vi "mHTprofile_vector.vi"(0 "Gamma0":dbl caption="Gamma0 (0)" format="%#_13g", 1 "Delta0":dbl caption="Delta0 (0)" format="%#_13g", 2 "Gamma2":dbl caption="Gamma2 (0)" format="%#_13g", 3 "Delta2":dbl caption="Delta2 (0)" format="%#_13g", 4 "NuOptRe":dbl caption="NuOptRe (0)" format="%#_13g", 5 "NuOptIm":dbl caption="NuOptIm (0)" format="%#_13g", 6 "Xlm":dbl caption="Xlm (0)" format="%#_13g", 7 "nu0":dbl caption="nu0 (0)" format="%#_13g", 8 "Ylm":dbl caption="Ylm (0)" format="%#_13g", 9 "GammaD":dbl caption="GammaD (0)" format="%#_13g", 10 "alpha":dbl=10.0 caption="alpha (10)" format="%#_13g", 11 "nu":dbl[](array[numeric])=[0.0, 112265.43344000001, 112265.44046000001, 112265.44748000002, 112265.45450000002, 112265.46152000003, 112265.46854000003, 112265.47556000004, 112265.48258000004, 112265.48960000004, 112265.49662000005, 112265.50364000005, 112265.51066000006, 112265.51768000006, 112265.52470000007, 112265.53172000007, 112265.53874000008, 112265.54576000008, 112265.55278000009, 112265.55980000009, 112265.5668200001, 112265.5738400001, 112265.5808600001, 112265.58788000011, 112265.59490000011, 112265.60192000012, 112265.60894000012, 112265.61596000013, 112265.62298000013, 112265.63000000014, 112265.63702000014, 112265.64404000014, 112265.65106000015, 112265.65808000015, 112265.66510000016, 112265.67212000016, 112265.67914000017, 112265.68616000017, 112265.69318000018, 112265.70020000018, 112265.70722000019, 112265.71424000019, 112265.7212600002, 112265.7282800002, 112265.7353000002, 112265.74232000021, 112265.74934000021, 112265.75636000022, 112265.76338000022, 112265.77040000023, 0.0] format="%#_16g", 12 "disp":enum32{"Absorption", "Dispersion"}(ring) caption="disp (Absorption)") -> (18 "mHT":dbl[](array[numeric])=[nan, 0.10445929269462101, 0.11168038230081595, 0.11969856238844125, 0.1286377380830614, 0.13864704864655428, 0.14990727829379918, 0.16263922460671215, 0.1771147209669791, 0.19367128964614844, 0.21273180576293013, 0.23483113593592242, 0.2606525606824893, 0.29107801057316474, 0.32725789462097354, 0.3707087581774661, 0.4234503518208136, 0.4881979797546625, 0.5686309274509256, 0.6697622885290168, 0.798437386757727, 0.9639839696835227, 1.1790249509999895, 1.460444698920676, 1.8304717689294367, 2.31776489642677, 2.9580972384622766, 3.7933109622015557, 4.86494935246605, 6.194795635571412, 7.740733853926797, 9.326488123304564, 10.59710374177369, 11.127748547057859, 10.714837692264172, 9.553864870950973, 8.06020224435464, 6.58240100721215, 5.295904040882446, 4.245577585161483, 3.4134497282314253, 2.761721832470126, 2.252063531475144, 1.8520390876765764, 1.5360968914463138, 1.2847114253118193, 1.0831306600151056, 0.9202283794901738, 0.7875855185711089, 0.6787942573273069, 1.4180731455680285e-09] caption="mHT output" format="%#_16g")   [LabVIEW 2015]
panel:
  # "modified Hartman Tran profile"
  # "Subroutine to compute the complex normalized spectral-line shape using mHT model\n\nStandard Input Parameters:\n--------------------\nnu0     : Unperturbed line position in cm-1.\nGammaD  : Doppler broadening in cm-1.\nGamma0  : Speed-averaged line-width in cm-1.       \nGamma2  : Quadratic speed dependence parameter of the line-width in cm-1.\nDelta0  : Speed-averaged line-shift in cm-1.\nDelta2  : Quadratic speed dependence parameter of the line-shift in cm-1.   \nNuOptRe : Real part of the complex Dicke parameter in cm-1.\nNuOptIm : Imaginary part of the complex Dicke parameter in cm-1.    \nnu      : Current WaveNumber in cm-1.\nYlm     : Imaginary part of the 1st order (Rosenkranz) line mixing coefficients, dimensionless (default: 0.0).\nXlm     : Real part of the 1st order (Rosenkranz) line mixing coefficients, dimensionless (default: 0.0).\nalpha   : Mass ratio in the molecule for calculating beta-correction, applicable up to alpha=5, \n          dimensionless (default: 10.0).\ndisp    : Boolean trigger for including dispersion profile in the output (default: Absorption).\n\nThe function has one outputs:\n--------------------\n(1)     : Real or imaginary (depending on disp value) part of the normalized spectral shape in cm."
  # "Output Section"
  # "Input Section"
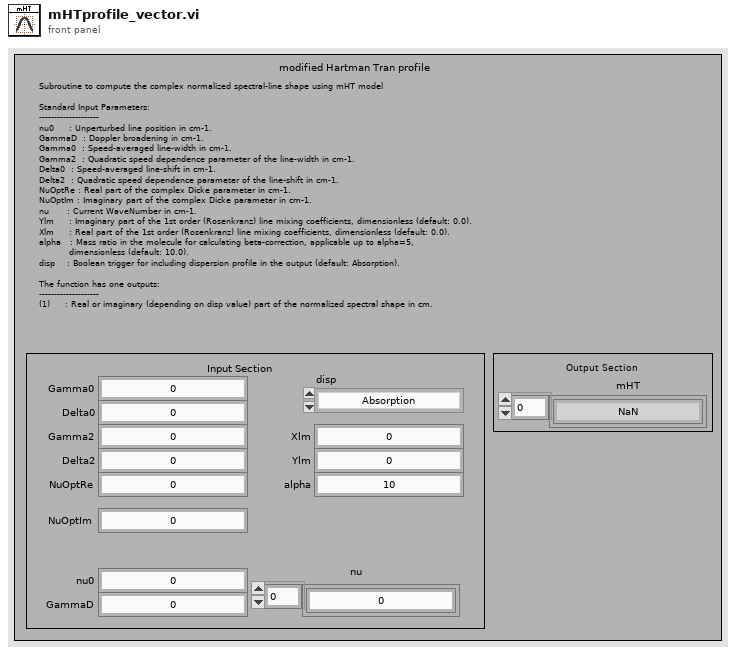
[diagram p1: front panel]
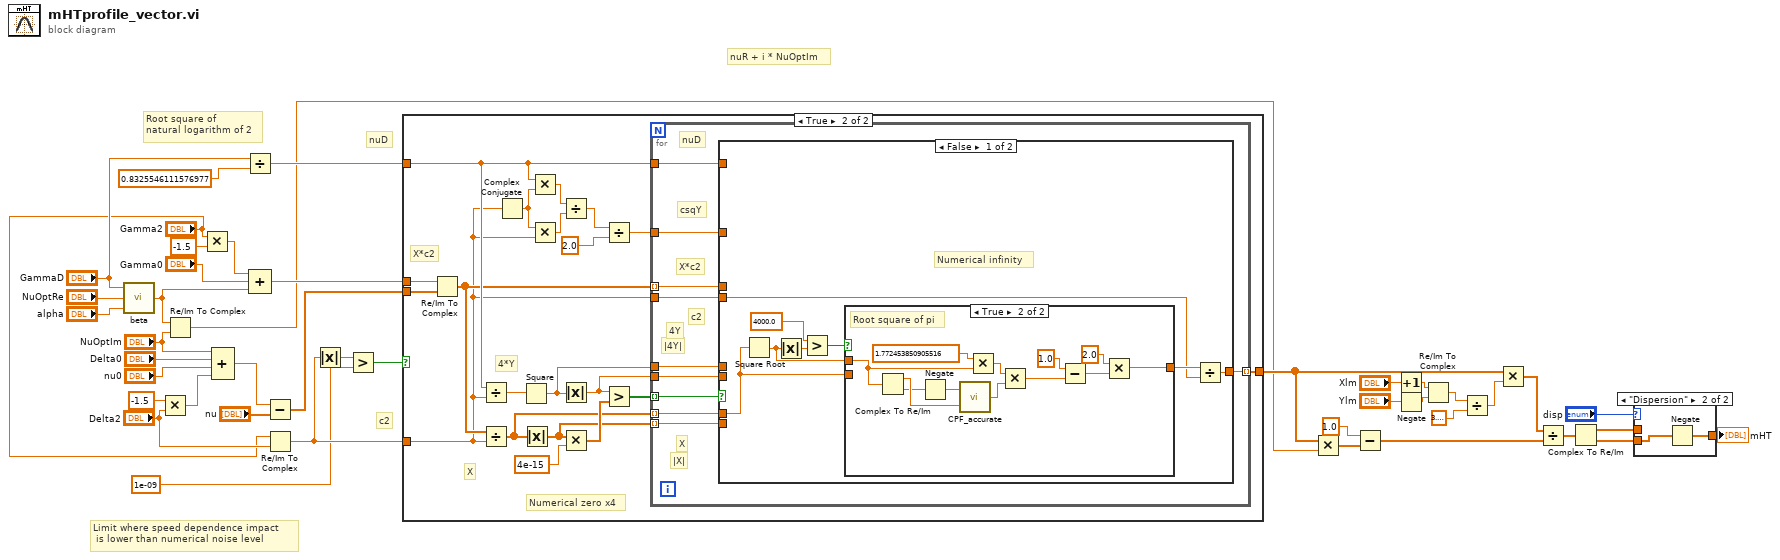
[diagram p0: block diagram]
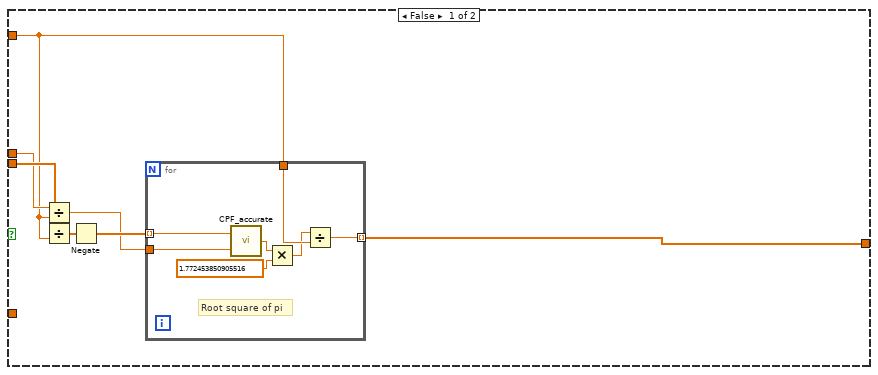
[diagram p3: hidden frame]
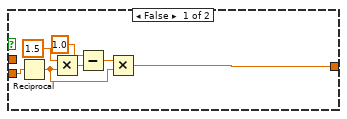
[diagram p4: hidden frame]
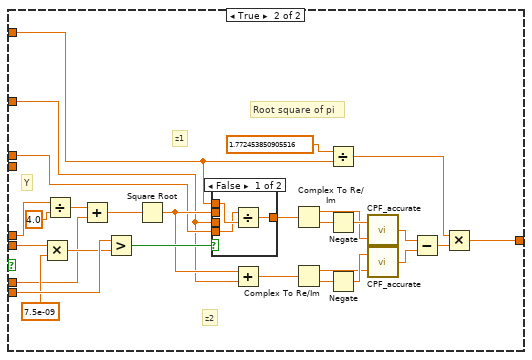
[diagram p5: hidden frame]
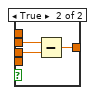
[diagram p6: hidden frame]
diagram:
  # "nuR + i * NuOptIm"
  # "nuD"
  # "c2"
  # "Limit where speed dependence impact\n is lower than numerical noise level"
  # "Root square of\nnatural logarithm of 2"
  n1 = call "beta.vi"("alpha"="alpha", "NuOptRe"="NuOptRe", "GammaD"="GammaD") -> ("nuR"=w13:dbl)
  n2 = Multiply(x=-1.5 ("y"), y="Delta2") -> (x*y=w5:dbl)
  n3 = Re/Im To Complex(1:"NuOptIm", 2:w13) -> (0:w27:cdb)
  n4 = Multiply(x="Gamma2", y=-1.5) -> (x*y=w12:dbl)
  n5 = Compound Arithmetic op=ADD("NuOptIm", "Delta0", "nu0", w5) -> (w4:dbl)
  n6 = Divide(x="GammaD", y=0.8325546111576977 ("sln2")) -> (x/y=w33:dbl)
  n7 = Compound Arithmetic op=ADD(w12, "Gamma0", w13) -> (w35:dbl)
  n8 = Subtract(x=w4, y="nu") -> (x-y=w34:dbl[])
  n9 = Re/Im To Complex(1:"Delta2", 2:"Gamma2") -> (0:w8:cdb)
  n10 = Absolute Value(x=w8) -> (abs(x)=w37:dbl)
  n11 = Greater?(x=w37, y=1e-09) -> (0:w36:bool)
  n12 = case shown="True" w36 {
    tunnel: w35 -> [w48 w76]
    tunnel: w34 -> [w49 w60]
    tunnel: w33 -> [w44 w61]
    tunnel: w8 -> [_ w58]
    tunnel: [w43 w62] -> w28
    frame False {
      n13 = Divide(x=w48, y=w44) -> (x/y=w45:dbl)
      n14 = Divide(x=w49, y=w44) -> (x/y=w47:dbl[])
      n15 = Negate(x=w47) -> (-x=w46:dbl[])
      n16 = for {
        tunnel: w46 -> [w56] mode=indexing
        tunnel: w45 -> [w55]
        tunnel: w44 -> [w52]
        tunnel: [w50] -> w43 mode=indexing
        # "Root square of pi"
        n17 = call "CPF_accurate.vi"("y"=w55, "x"=w56) -> ("CPF Value"=w54:cdb)
        n18 = Multiply(x=w54, y=1.772453850905516) -> (x*y=w51:cdb)
        n19 = Divide(x=w51, y=w52) -> (x/y=w50:cdb)
      }
    }
    frame True {
      # "4*Y"
      # "X"
      # "X*c2"
      # "Numerical zero x4"
      n20 = Re/Im To Complex(1:w60, 2:w76) -> (0:w59:cdb[])
      n21 = Divide(x=w61, y=w58) -> (x/y=w75:cdb)
      n22 = Divide(x=w59, y=w58) -> (x/y=w66:cdb[])
      n23 = Complex Conjugate(1:w58) -> (0:w72:cdb)
      n24 = Square(x=w75) -> (x^2=w65:cdb)
      n25 = Absolute Value(x=w66) -> (abs(x)=w64:dbl[])
      n26 = Multiply(x=w61, y=w72) -> (x*y=w71:cdb)
      n27 = Multiply(x=w72, y=w58) -> (x*y=w70:cdb)
      n28 = Divide(x=w71, y=w70) -> (x/y=w69:cdb)
      n29 = Absolute Value(x=w65) -> (abs(x)=w63:dbl)
      n30 = Multiply(x=w64, y=4e-15 ("sln2")) -> (x*y=w74:dbl[])
      n31 = Divide(x=w69, y=2.0) -> (x/y=w67:cdb)
      n32 = Greater?(x=w63, y=w74) -> (0:w73:bool[])
      n33 = for {
        tunnel: w73 -> [w86] mode=indexing
        tunnel: w67 -> [w85]
        tunnel: w66 -> [w84] mode=indexing
        tunnel: w65 -> [w83]
        tunnel: w64 -> [w82] mode=indexing
        tunnel: w63 -> [w81]
        tunnel: [w80] -> w62 mode=indexing
        tunnel: w61 -> [w79]
        tunnel: w59 -> [w78] mode=indexing
        tunnel: w58 -> [w77]
        # "|4Y|"
        # "4Y"
        # "|X|"
        # "X"
        # "c2"
        # "X*c2"
        # "csqY"
        # "nuD"
        n34 = case shown="False" w86 {
          tunnel: w85 -> [_ w115]
          tunnel: w84 -> [w91 w129]
          tunnel: w77 -> [w93 _]
          tunnel: w83 -> [_ w138]
          tunnel: w82 -> [_ w133]
          tunnel: w81 -> [_ w132]
          tunnel: w78 -> [_ w116]
          tunnel: w79 -> [_ w114]
          tunnel: [w87 w117] -> w80
          frame False {
            # "Numerical infinity"
            n35 = Square Root(x=w91) -> (sqrt(x)=w88:cdb)
            n36 = Absolute Value(x=w88) -> (abs(x)=w92:dbl)
            n37 = Greater?(x=4000.0 ("sln2"), y=w92) -> (0:w89:bool)
            n38 = case shown="True" w89 {
              tunnel: w91 -> [w101 _]
              tunnel: w88 -> [_ w102]
              tunnel: [w96 w103] -> w94
              frame False {
                n39 = Reciprocal(x=w101) -> (1/x=w95:cdb)
                n40 = Multiply(x=1.5, y=w95) -> (x*y=w99:cdb)
                n41 = Subtract(x=1.0, y=w99) -> (x-y=w97:cdb)
                n42 = Multiply(x=w97, y=w95) -> (x*y=w96:cdb)
              }
              frame True {
                # "Root square of pi"
                n43 = Complex To Re/Im(x + iy=w102) -> (x=w112:dbl, y=w111:dbl)
                n44 = Negate(x=w111) -> (-x=w113:dbl)
                n45 = call "CPF_accurate.vi"("y"=w112, "x"=w113) -> ("CPF Value"=w109:cdb)
                n46 = Multiply(x=1.772453850905516, y=w102) -> (x*y=w108:cdb)
                n47 = Multiply(x=w108, y=w109) -> (x*y=w107:cdb)
                n48 = Subtract(x=1.0, y=w107) -> (x-y=w105:cdb)
                n49 = Multiply(x=2.0, y=w105) -> (x*y=w103:cdb)
              }
            }
            n50 = Divide(x=w94, y=w93) -> (x/y=w87:cdb)
          }
          frame True {
            # "z2"
            # "z1"
            # "Y"
            # "Root square of pi"
            n51 = Multiply(x=w132, y=7.5e-09) -> (x*y=w130:dbl)
            n52 = Divide(x=w138, y=4.0) -> (x/y=w140:cdb)
            n53 = Add(x=w140, y=w129) -> (x+y=w141:cdb)
            n54 = Greater?(x=w133, y=w130) -> (0:w137:bool)
            n55 = Square Root(x=w141) -> (sqrt(x)=w135:cdb)
            n56 = case shown="False" w137 {
              tunnel: w135 -> [_ w147]
              tunnel: w115 -> [_ w146]
              tunnel: [w143 w145] -> w136
              tunnel: w114 -> [w144 _]
              tunnel: w116 -> [w142 _]
              frame False {
                n57 = Divide(x=w142, y=w144) -> (x/y=w143:cdb)
              }
              frame True {
                n58 = Subtract(x=w147, y=w146) -> (x-y=w145:cdb)
              }
            }
            n59 = Add(x=w135, y=w115) -> (x+y=w134:cdb)
            n60 = Complex To Re/Im(x + iy=w136) -> (x=w123:dbl, y=w126:dbl)
            n61 = Complex To Re/Im(x + iy=w134) -> (x=w124:dbl, y=w125:dbl)
            n62 = Divide(x=1.772453850905516, y=w114) -> (x/y=w118:dbl)
            n63 = Negate(x=w126) -> (-x=w128:dbl)
            n64 = Negate(x=w125) -> (-x=w127:dbl)
            n65 = call "CPF_accurate.vi"("y"=w123, "x"=w128) -> ("CPF Value"=w122:cdb)
            n66 = call "CPF_accurate.vi"("y"=w124, "x"=w127) -> ("CPF Value"=w121:cdb)
            n67 = Subtract(x=w122, y=w121) -> (x-y=w119:cdb)
            n68 = Multiply(x=w118, y=w119) -> (x*y=w117:cdb)
          }
        }
      }
    }
  }
  n69 = Multiply(x=w28, y=w27) -> (x*y=w25:cdb[])
  n70 = Subtract(x=1.0, y=w25) -> (x-y=w23:cdb[])
  n71 = Increment(x="Xlm") -> (x+1=w31:dbl)
  n72 = Negate(x="Ylm") -> (-x=w2:dbl)
  n73 = Re/Im To Complex(1:w2, 2:w31) -> (0:w30:cdb)
  n74 = Divide(x=w30, y=3.141592653589793) -> (x/y=w29:cdb)
  n75 = Multiply(x=w28, y=w29) -> (x*y=w24:cdb[])
  n76 = Divide(x=w24, y=w23) -> (x/y=w22:cdb[])
  n77 = Complex To Re/Im(x + iy=w22) -> (x=w20:dbl[], y=w19:dbl[])
  n78 = case shown="\"Dispersion\"" "disp" {
    tunnel: w20 -> [w148 _]
    tunnel: w19 -> [_ w150]
    tunnel: [w148 w149] -> w18
    frame "Absorption", Default {
    }
    frame "Dispersion" {
      n79 = Negate(x=w150) -> (-x=w149:dbl[])
    }
  }
  "mHT" <- w18
